vi "Initialize Thread.vi"(8 "error in (no error)":errorcluster, 10 "thread settings":T1[](array[typedef]), 11 "UDP Transceiver in":refnum<class "UDP Transceiver.lvclass">) -> (0 "error out":errorcluster, 3 "UDP Transceiver out":refnum<class "UDP Transceiver.lvclass">)   [LabVIEW 2017, in "DSF Core.lvlib" / "UDP Transceiver.lvclass"]
uses:
  UDP Transceiver.lvclass
  Typedefs/DSF Settings Info.ctl
  Typedefs/DSF Version Info.ctl
  UDP Transceiver.lvclass/UDP Transceiver.ctl
  Throw Unknown Setting Error.vi
  Classes/Configuration Session/Configuration Session.lvclass
  DSF Core.lvlib
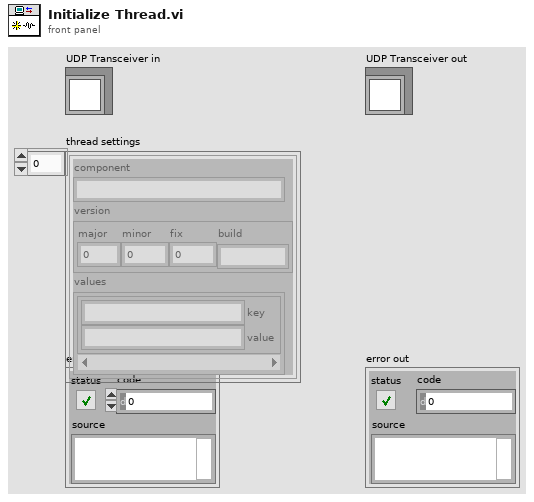
[diagram p1: front panel]
types:
  T1 = typedef "DSF Core.lvlib/DSF Settings Info.ctl" = cluster{"component":string, "version":T2, "values":cluster{"key":string, "value":string}[]}
  T2 = typedef "DSF Core.lvlib/DSF Version Info.ctl" = cluster{"major":u32, "minor":u32, "fix":u32, "build":string}
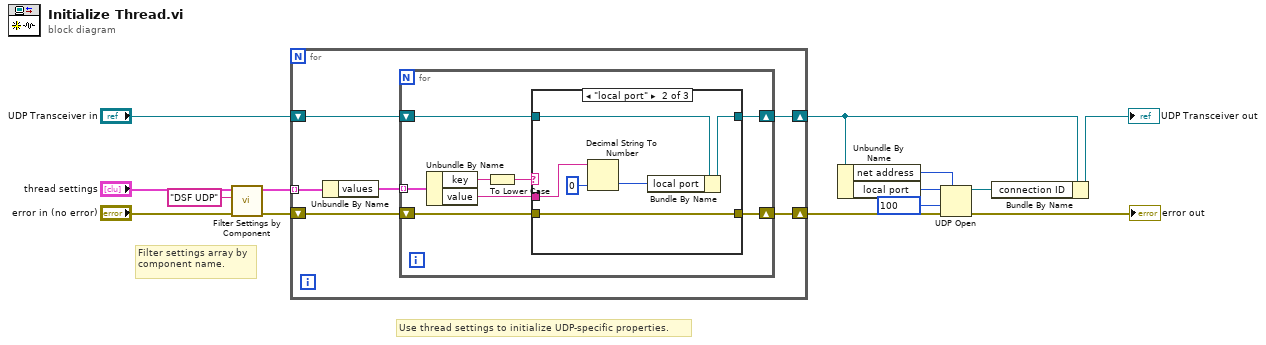
[diagram p0: block diagram]
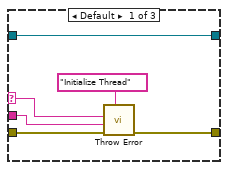
[diagram p2: hidden frame]
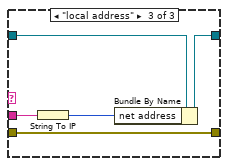
[diagram p3: hidden frame]
diagram:
  # "Filter settings array by component name."
  # "Use thread settings to initialize UDP-specific properties."
  n1 = call "Filter Settings by Component.vi"("error in (no error)"="error in (no error)", "component"="DSF UDP", "settings"="thread settings") -> ("error out"=w12:errorcluster, "filtered settings"=w14:T1[])  [unwired: 7 in]
  n2 = for {
    tunnel: w14 -> [w16] mode=indexing
    shift-right: [w19] -> w2
    shift-left: "UDP Transceiver in" -> [w20]
    shift-right: [w17] -> w4
    shift-left: w12 -> [w18]
    n3 = Unbundle By Name(w16) -> ("values"=w15:cluster{"key":string, "value":string}[])
    n4 = for {
      shift-right: [w27] -> w19
      shift-left: w20 -> [w28]
      shift-right: [w25] -> w17
      shift-left: w18 -> [w26]
      tunnel: w15 -> [w24] mode=indexing
      n5 = Unbundle By Name(w24) -> ("key"=w22:string, "value"=w23:string)
      n6 = To Lower Case(string=w22) -> (all lower case string=w21:string)
      n7 = case shown="\"local port\"" w21 {
        selector: w21 -> [w32 _ _]
        tunnel: w28 -> [w29 w35 w45]
        tunnel: [w29 w39 w44] -> w27
        tunnel: w26 -> [w34 w38 w43]
        tunnel: [w33 w38 w43] -> w25
        tunnel: w23 -> [w30 w36 w41]
        frame Default {
          n8 = call-poly "Throw Error.vi"("source vi name"="Initialize Thread", "error in (no error)"=w34, "value"=w30, "key"=w32) -> ("error out"=w33:errorcluster)  [unwired: 7 in]
        }
        frame "local port" {
          n9 = Decimal String To Number(string=w36, default (0L)=u16 0 ("default (0 I32)")) -> (number=w37:u16)  [unwired: 1 in, 1 out]
          n10 = Bundle By Name(cluster=w35, "local port"=w37) -> (w39:refnum<class "UDP Transceiver.lvclass">)
        }
        frame "local address" {
          n11 = String To IP(1:w41) -> (0:w42:u32)
          n12 = Bundle By Name(cluster=w45, "net address"=w42) -> (w44:refnum<class "UDP Transceiver.lvclass">)
        }
      }
    }
  }
  n13 = Unbundle By Name(w2) -> ("net address"=w5:u32, "local port"=w8:u16)
  n14 = UDP Open(7:w5, 8:w4, 9:100 ("timeout ms (25000)"), 11:w8) -> (port=w6:refnum<k16>, 0:→"error out":errorcluster)  [unwired: 1 in, 1 out]
  n15 = Bundle By Name(cluster=w2, "connection ID"=w6) -> (→"UDP Transceiver out":refnum<class "UDP Transceiver.lvclass">)
